vi "Settings.vi"(8 "error in (no error)":errorcluster, 11 "Settings In":T1) -> (0 "error out":errorcluster, 3 "Settings Out":T1)   [LabVIEW 2020]
uses:
  Settings/Settings.ctl
  controls/Hardware Configuration.ctl
  Logging/Logging Configuration.ctl
  Acquisition/Acquisition.lvlib
  Logging/Logging.lvlib
  Settings/Settings.lvlib
panel:
  in  "Samples to Log":u32=500 min=1
  in  "Log File Path":path=path "C:/Users/Conner/OneDrive - University of Louisville/Documents/Labview logging test"
  in  "DAQmx Task":refnum<k21>="Sim AI Task"
  in  "OK Button":bool
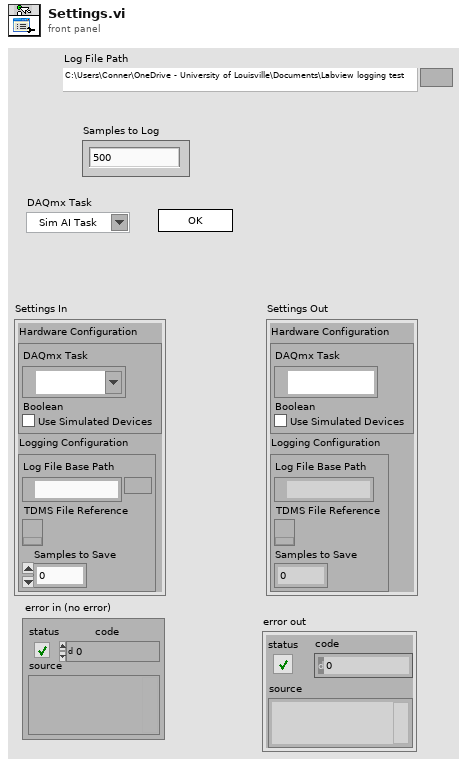
[diagram p1: front panel]
types:
  T1 = typedef "Settings.lvlib/Settings.ctl" = cluster{"Hardware Configuration":T2, "Logging Configuration":T3}
  T2 = typedef "Acquisition.lvlib/Hardware Configuration.ctl" = cluster{"DAQmx Task":refnum<k21>, "Boolean":bool}
  T3 = typedef "Logging.lvlib/Logging Configuration.ctl" = cluster{"Log File Base Path":path, "TDMS File Reference":refnum<k34>, "Samples to Save":u32}
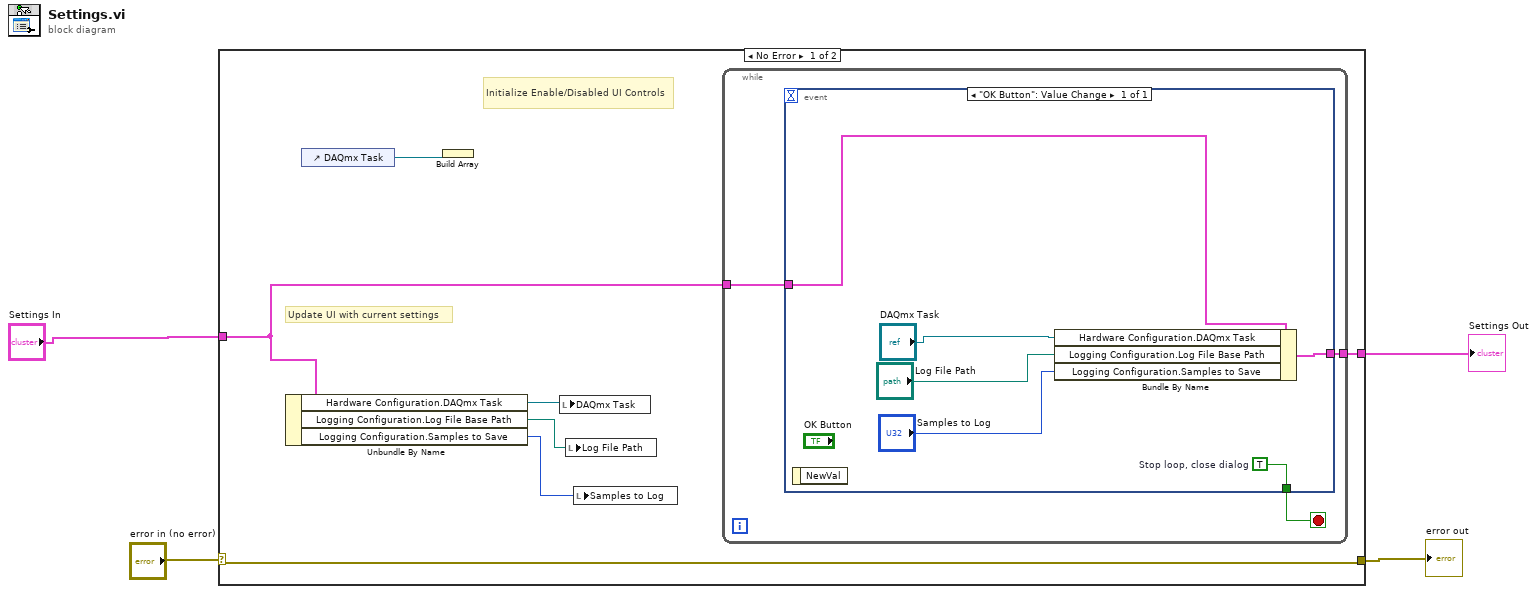
[diagram p0: block diagram]
diagram:
  n1 = case shown="No Error" "error in (no error)" {
    selector: "error in (no error)" -> [w11 w22]
    tunnel: [w11 w22] -> w3
    tunnel: "Settings In" -> [w8 w21]
    tunnel: [w10 w21] -> w1
    frame No Error {
      # "Initialize Enable/Disabled UI Controls"
      # "Update UI with current settings"
      n2 = Unbundle By Name(w8) -> ("Hardware Configuration.DAQmx Task"=w7:refnum<k21>, "Logging Configuration.Log File Base Path"=w6:path, "Logging Configuration.Samples to Save"=w5:u32)
      n3 = control-ref of="DAQmx Task"() -> (w9:refnum<vi>)
      n4 = Build Array(w9) -> ()  [unwired: 1 out]
      n5 = local write "DAQmx Task"(w7) -> ()
      n6 = local write "Log File Path"(w6) -> ()
      n7 = local write "Samples to Log"(w5) -> ()
      n8 = while {
        tunnel: w8 -> [w13]
        tunnel: [w12] -> w10
        stop <- w14 stop-if-true
        n9 = event shown="[0] \"OK Button\": Value Change" {
          selector: _ -> [_]
          dyn-events: _ -> [_]
          timeout: _ -> [_]
          tunnel: [w20] -> w14
          tunnel: w13 -> [w19]
          tunnel: [w15] -> w12
          event "OK Button": Value Change {
            w20 = TRUE  # Stop loop, close dialog
            n10 = event-data() -> ()  [unwired: 1 in, 1 out]
            n11 = Bundle By Name(cluster=w19, "Hardware Configuration.DAQmx Task"="DAQmx Task", "Logging Configuration.Log File Base Path"="Log File Path", "Logging Configuration.Samples to Save"="Samples to Log") -> (w15:T1)
          }
        }
      }
    }
    frame Error {
    }
  }
  "error out" <- w3
  "Settings Out" <- w1
